vi "文件列表 2.vi"() -> ()   [LabVIEW 2023]
panel:
  in  "Listbox 4":i32(listbox)
  in  "Listbox 3":i32(listbox)
  out "element":string
  in  "stop":bool
  in  "Listbox 2":i32(listbox)
  in  "Listbox":i32[](listbox)
  in  "Ring":u16(ring) items=["monday", "tuesday", "wednesday"]
  # "文件列表 2"
  # "Example 1"
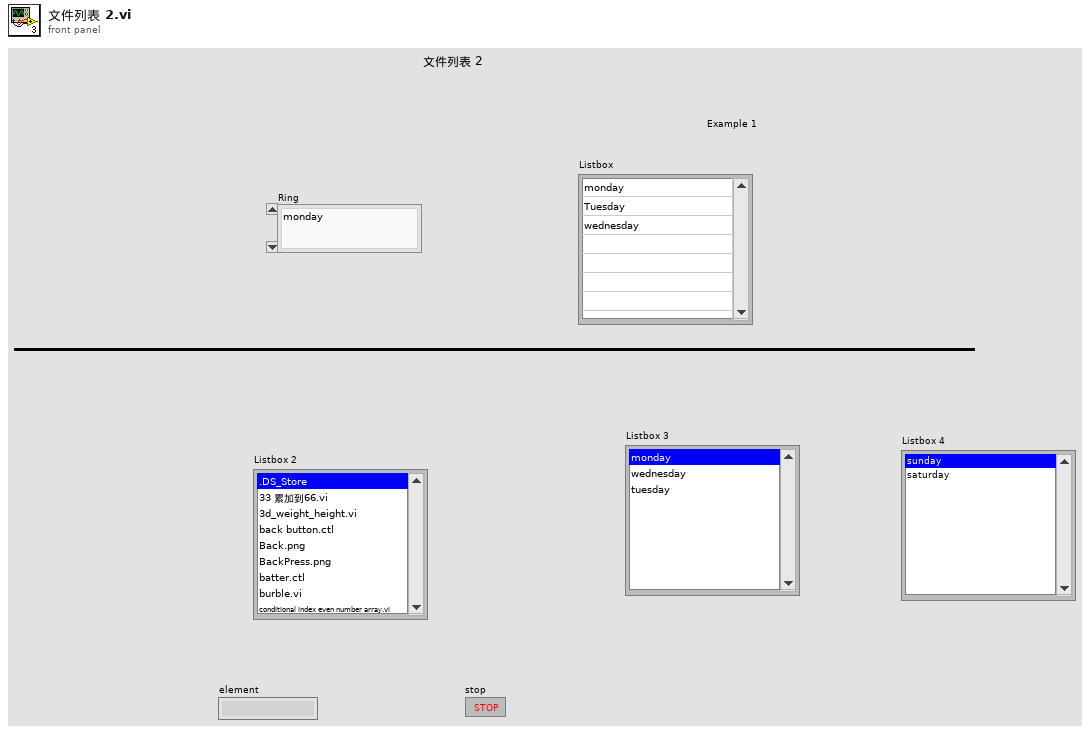
[diagram p1: front panel]
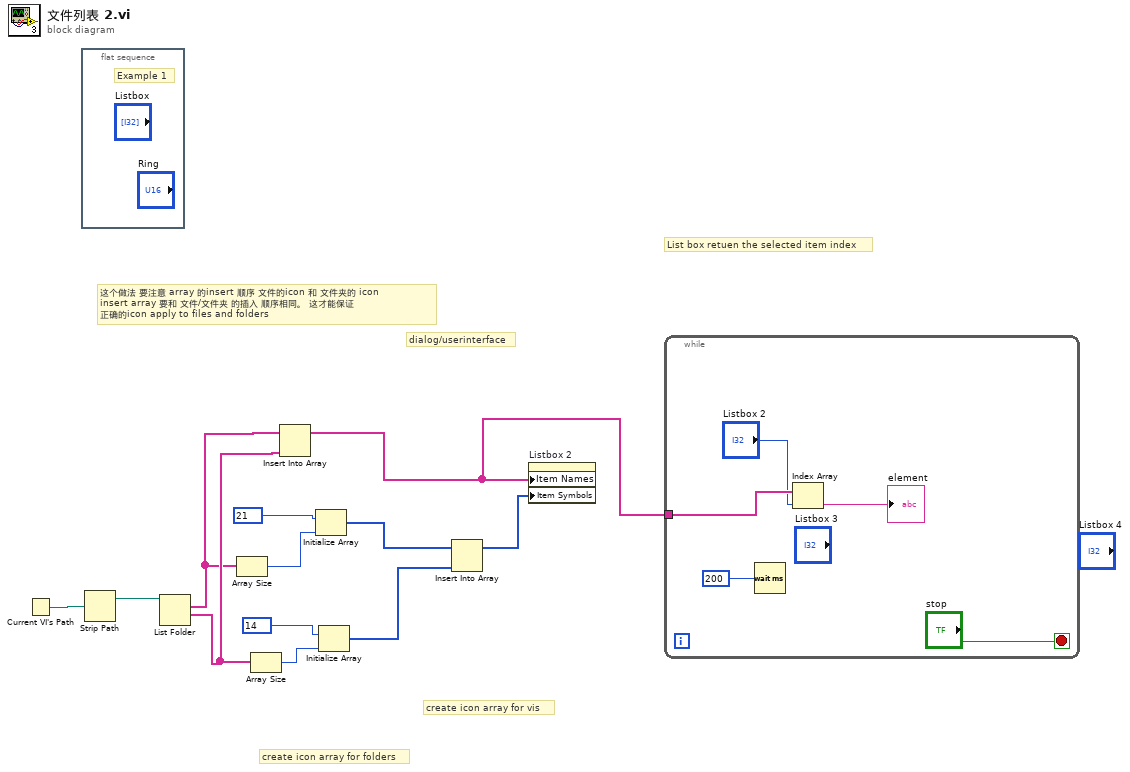
[diagram p0: block diagram]
diagram:
  # "create icon array for folders"
  # "create icon array for vis"
  # "List box retuen the selected item index"
  # "这个做法 要注意 array 的insert 顺序 文件的icon 和 文件夹的 icon \ninsert array 要和 文件/文件夹 的插入 顺序相同。 这才能保证\n正确的icon apply to files and folders"
  # "dialog/userinterface"
  n1 = Current VI's Path() -> (path=w12:path)
  n2 = flat-sequence {
    frame #0 {
      # "Example 1"
    }
  }
  n3 = Strip Path(path=w12) -> (stripped path=w11:path)  [unwired: 1 out]
  n4 = List Folder(path=w11) -> (filenames=w1:string[], folder names=w3:string[])  [unwired: 3 in, 2 out]
  n5 = Array Size(array=w1) -> (size(s)=w10:i32)
  n6 = Array Size(array=w3) -> (size(s)=w8:i32)
  n7 = Insert Into Array "Insert Into Array"(array=w1, new element=w3) -> (w2:string[])  [unwired: 1 in]
  n8 = Initialize Array "Initialize Array"(21, w10) -> (w6:i32[])
  n9 = Initialize Array "Initialize Array"(14, w8) -> (w5:i32[])
  n10 = Insert Into Array "Insert Into Array"(array=w6, new element=w5) -> (w4:i32[])  [unwired: 1 in]
  n11 = property on="Listbox 2" class="LstBox (strict)"("Item Names"=w2, "Item Symbols"=w4) -> ()  [unwired: 2 in, 2 out]
  n12 = while {
    tunnel: w2 -> [w17]
    stop <- "stop" stop-if-true
    n13 = Wait (ms)(milliseconds to wait=u32 200) -> ()  [unwired: 1 out]
    n14 = Index Array "Index Array"(array=w17, index="Listbox 2") -> (element=→"element":string)
  }
